vi "Linear Fit Coefficients.vi"(0 "Y":dbl[](array[numeric]), 5 "X":dbl[](array[numeric]), 7 "Weight":dbl[](array[numeric]), 9 "tolerance":dbl=0.0001, 11 "method":T1 items=["Least Square", "Least Absolute Residual", "Bisquare"]) -> (4 "slope":dbl, 6 "intercept":dbl, 15 "error":i32)   [LabVIEW 2010, in "NI_AALPro.lvlib"]
doc: "Returns the <B>slope</B> and <B>intercept</B> of the linear fit for a data set (<B>X</B>, <B>Y</B>) using the Least Square, Least Absolute Residual, or Bisquare method."
uses:
  NI_AALPro.lvlib
  Curve Fitting Criteria.ctl
panel:
  # "Linear Fit Coefficients"
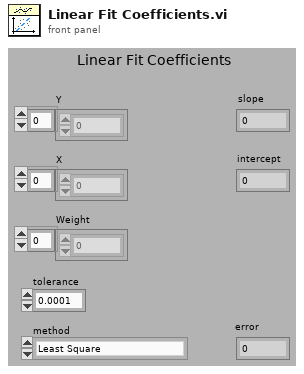
[diagram p1: front panel]
types:
  T1 = typedef "NI_AALPro.lvlib/Curve Fitting Criteria.ctl" = u16
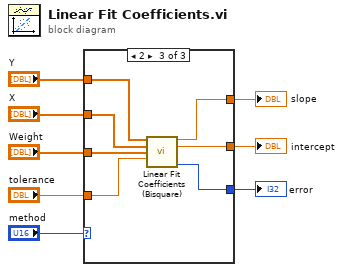
[diagram p0: block diagram]
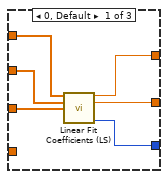
[diagram p2: hidden frame]
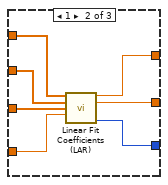
[diagram p3: hidden frame]
diagram:
  n1 = case shown="2" "method" {
    tunnel: "Y" -> [w14 w21 w28]
    tunnel: "X" -> [w13 w20 w27]
    tunnel: "Weight" -> [w12 w19 w26]
    tunnel: [w11 w17 w24] -> w4
    tunnel: [w10 w16 w23] -> w3
    tunnel: [w9 w15 w22] -> w2
    tunnel: "tolerance" -> [_ w18 w25]
    frame 0, Default {
      n2 = call "Linear Fit Coefficients (LS).vi"("Y"=w14, "X"=w13, "Weight"=w12) -> ("slope"=w11:dbl, "intercept"=w10:dbl, "error"=w9:i32)  [unwired: 10 out]
    }
    frame 1 {
      n3 = call "Linear Fit Coefficients (LAR).vi"("Y"=w21, "X"=w20, "Weight"=w19, "tol"=w18) -> ("slope"=w17:dbl, "intercept"=w16:dbl, "error"=w15:i32)  [unwired: 9 out]
    }
    frame 2 {
      n4 = call "Linear Fit Coefficients (Bisquare).vi"("Y"=w28, "X"=w27, "Weight"=w26, "tol"=w25) -> ("slope"=w24:dbl, "intercept"=w23:dbl, "error"=w22:i32)  [unwired: 9 out]
    }
  }
  "slope" <- w4
  "intercept" <- w3
  "error" <- w2
